vi "close connection.vi"(8 "error in (no error)":errorcluster, 11 "OHAUS_232 in":refnum<class "OHAUS_Navigator_232.lvclass">) -> (0 "error out":errorcluster, 3 "OHAUS_232 out":refnum<class "OHAUS_Navigator_232.lvclass">)   [LabVIEW 2019, in "OHAUS_Navigator_232.lvclass"]
uses:
  OHAUS_Navigator_232.lvclass
  OHAUS_Navigator_232.lvclass/OHAUS_Navigator_232.ctl
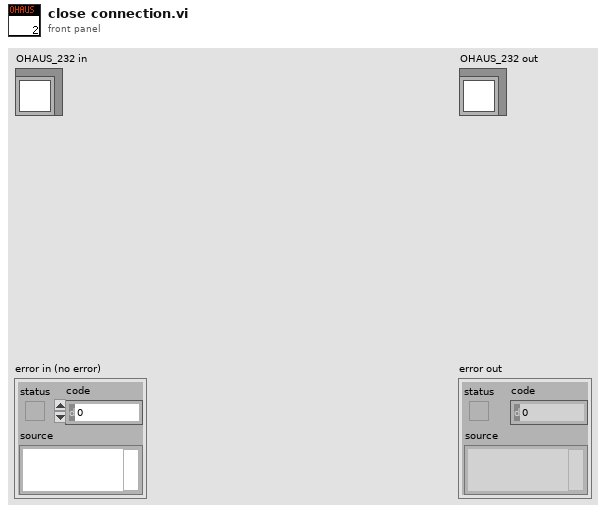
[diagram p1: front panel]
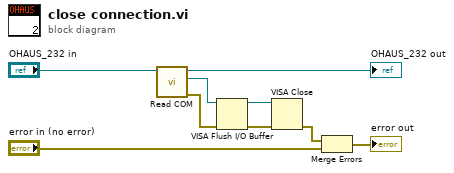
[diagram p0: block diagram]
diagram:
  n1 = call "Read COM.vi"("OHAUS_232 in"="OHAUS_232 in") -> ("error out"=w5:errorcluster, "COM"=w6:refnum<visa-resource-name>, "OHAUS_232 out"=→"OHAUS_232 out":refnum<class "OHAUS_Navigator_232.lvclass">)  [unwired: 8 in]
  n2 = VISA Flush I/O Buffer(VISA resource name=w6, error in (no error)=w5) -> (VISA resource name out=w4:refnum<visa-resource-name>, error out=w3:errorcluster)  [unwired: 1 in]
  n3 = VISA Close(VISA resource name=w4, error in (no error)=w3) -> (error out=w9:errorcluster)
  n4 = Merge Errors(w9, "error in (no error)") -> (→"error out":errorcluster)
